vi "subpanel (tsc).vi"   [LabVIEW 2018]
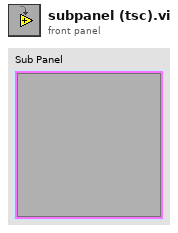
[diagram p1: front panel]
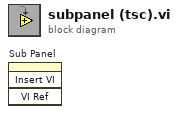
[diagram p0: block diagram]
diagram:
  n1 = invoke on="Sub Panel" class="SubPnl" method="Insert VI"() -> ()  [unwired: 4 in, 4 out]
